vi "Variant_to_Refnum.vi"(8 "Error in":errorcluster, 11 "Value (in)":variant) -> (0 "Error out":errorcluster, 2 "Value (string)":string, 3 "Value (out)":refnum<vi>, 5 "DAQmx Task Name":refnum<k21>, 7 "Image Dst Out":T1)   [LabVIEW 2012]
uses:
  <vilib>/vision/Image Controls.llb/IMAQ Image.ctl
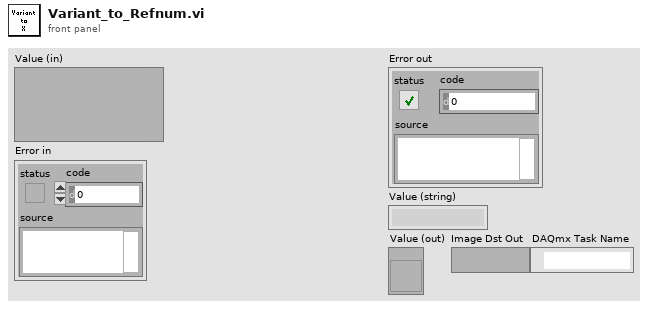
[diagram p1: front panel]
types:
  T1 = typedef "IMAQ Image.ctl" = refnum<image>
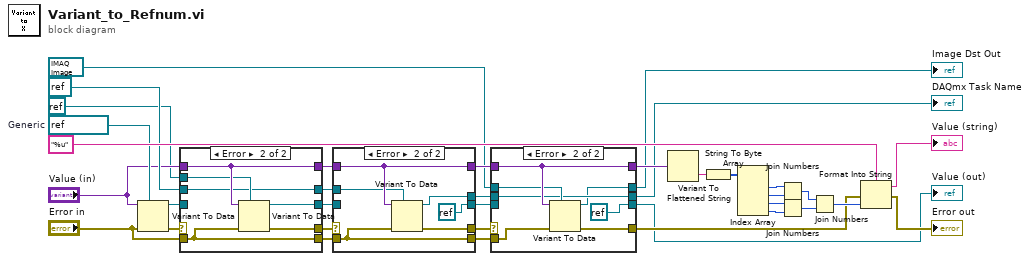
[diagram p0: block diagram]
diagram:
  w23 = refnum<vi> refnum  # Generic
  n1 = Variant To Data(error in="Error in", type=w23, Variant="Value (in)") -> (data=w9:refnum<vi>, error out=w8:errorcluster)
  n2 = case shown="Error" w8 {
    selector: w8 -> [w39 _]
    tunnel: w9 -> [w40 _]
    tunnel: [w40 w43] -> w11
    tunnel: [w39 w45] -> w12
    tunnel: [w38 w46] -> w10
    tunnel: "Value (in)" -> [w38 w46]
    tunnel: refnum<k21> refnum ("DAQmx Task Name") -> [w37 w42]
    tunnel: refnum<k0> refnum -> [_ w44]
    tunnel: [w37 w42] -> w4
    tunnel: "Error in" -> [w36 w41]
    tunnel: [w36 w41] -> w2
    frame No Error {
    }
    frame Error {
      n3 = Variant To Data(error in=w41, type=w44, Variant=w46) -> (data=w43:refnum<k0>, error out=w45:errorcluster)
    }
  }
  n4 = case shown="Error" w12 {
    selector: w12 -> [w50 _]
    tunnel: w11 -> [w51 _]
    tunnel: [w51 refnum<k0> refnum] -> w21
    tunnel: [w50 w55] -> w22
    tunnel: [w49 w57] -> w19
    tunnel: w10 -> [w49 w57]
    tunnel: w4 -> [w48 w56]
    tunnel: [w48 w54] -> w20
    tunnel: w2 -> [w47 w52]
    tunnel: [w47 w52] -> w1
    frame No Error {
    }
    frame Error {
      n5 = Variant To Data(error in=w52, type=w56, Variant=w57) -> (data=w54:refnum<k21>, error out=w55:errorcluster)
    }
  }
  n6 = case shown="Error" w22 {
    selector: w22 -> [w61 _]
    tunnel: w21 -> [w62 _]
    tunnel: [w62 refnum<k0> refnum] -> w15
    tunnel: [w61 w67] -> w16
    tunnel: [w59 w69] -> w18
    tunnel: w19 -> [w59 w69]
    tunnel: T1 refnum ("Image Dst Out") -> [w58 w68]
    tunnel: [w60 w65] -> w13
    tunnel: w20 -> [w60 w65]
    tunnel: [w58 w64] -> w14
    tunnel: w1 -> [_ w63]
    frame No Error {
    }
    frame Error {
      n7 = Variant To Data(error in=w63, type=w68, Variant=w69) -> (data=w64:T1, error out=w67:errorcluster)
    }
  }
  "Value (out)" <- w15
  "Image Dst Out" <- w14
  "DAQmx Task Name" <- w13
  n8 = Variant To Flattened String(Variant=w18) -> (data string=w35:string)  [unwired: 1 out]
  n9 = String To Byte Array(string=w35) -> (unsigned byte array=w34:u8[])
  n10 = Index Array(array=w34) -> (element #1=w33:u8, element #2=w32:u8, element #3=w31:u8, element #4=w30:u8)  [unwired: 4 in]
  n11 = Join Numbers(hi=w33, lo=w32) -> ((hi.lo)=w29:u16)
  n12 = Join Numbers(hi=w31, lo=w30) -> ((hi.lo)=w28:u16)
  n13 = Join Numbers(hi=w29, lo=w28) -> ((hi.lo)=w24:u32)
  n14 = Format Into String(format string="%u", error in=w16, w24) -> (resulting string=→"Value (string)":string, error out=→"Error out":errorcluster)  [unwired: 1 in]
